vi "plot.vi"(0 "reference":refnum<class "OSA.lvclass">, 3 "dataType":T1=enum."interferogram", 5 "error in (no error)":errorcluster, 9 "autoScale Y":bool) -> (14 "duplicate reference":refnum<class "OSA.lvclass">, 19 "error out":errorcluster)   [LabVIEW 2010, in "OSA.lvclass"]
doc: "This will write a plot in an intensity graph if a corresponding reference has been provided/routed to init.vi. A compatible graph to copy can be found in the tree.vi."
uses:
  OSA.lvclass
  OSA20X_misc.lvlib
  typeDef/acq_dataType.ctl
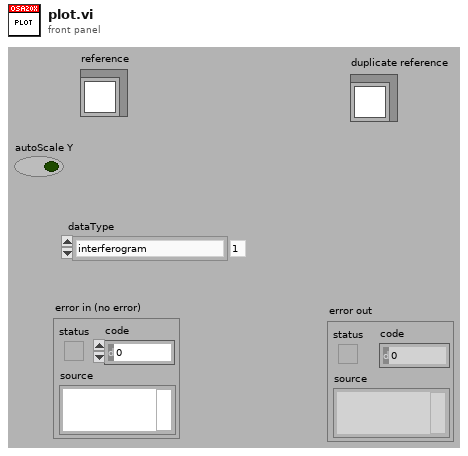
[diagram p1: front panel]
types:
  T1 = typedef "OSA.lvclass/acq_dataType.ctl" = enum16{"none", "interferogram", "spectrum"}
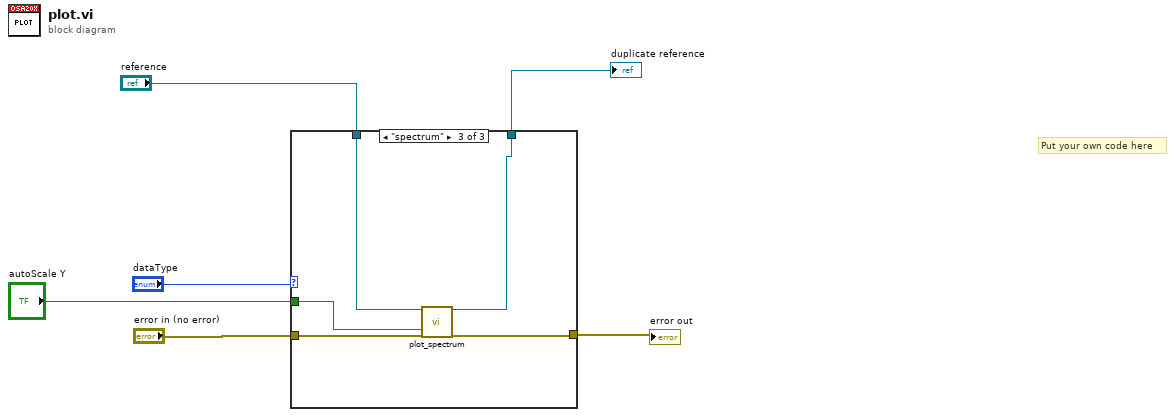
[diagram p0: block diagram]
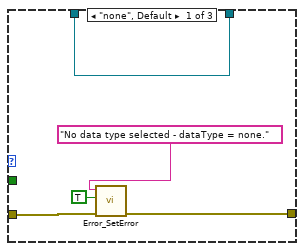
[diagram p2: hidden frame]
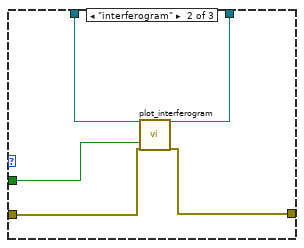
[diagram p3: hidden frame]
diagram:
  # "Put your own code here"
  n1 = case shown="\"spectrum\"" "dataType" {
    tunnel: "reference" -> [w7 w15 w19]
    tunnel: [w7 w14 w18] -> w6
    tunnel: "error in (no error)" -> [w9 w16 w21]
    tunnel: [w8 w13 w20] -> w1
    tunnel: "autoScale Y" -> [_ w12 w17]
    frame "none", Default {
      n2 = call "Error_SetError.vi"("error in"=w9, "status (true)"=TRUE, "source(\"\")"="No data type selected - dataType = none." ("source(\"\")")) -> ("error out"=w8:errorcluster)  [unwired: 4 in]
    }
    frame "interferogram" {
      n3 = call "plot_interferogram.vi"("reference"=w15, "autoScale Y"=w12, "error in (no error)"=w16) -> ("duplicate reference"=w14:refnum<class "OSA.lvclass">, "error out"=w13:errorcluster)  [unwired: 15 in]
    }
    frame "spectrum" {
      n4 = call "plot_spectrum.vi"("reference"=w19, "autoScale Y"=w17, "error in (no error)"=w21) -> ("duplicate reference"=w18:refnum<class "OSA.lvclass">, "error out"=w20:errorcluster)  [unwired: 15 in]
    }
  }
  "error out" <- w1
  "duplicate reference" <- w6
